vi "Handle Error.vi"(8 "error in (no error)":errorcluster, 11 "uService Template in":refnum<class "Father of all uServices.lvclass">) -> (0 "error out":errorcluster, 2 "stop actor?":bool=TRUE, 3 "uService Template out":refnum<class "Father of all uServices.lvclass">)   [LabVIEW 2026, in "TALOS.lvlib" / "Father of all uServices.lvlib" / "Father of all uServices.lvclass"]
doc: "(<B>Filename</B>: Actor Framework.lvlib:Actor.lvclass:Handle Error.vi)\n\nDefines how the actor handles an error that occurred while processing a message. By default, this method does nothing except stop the actor."
uses:
  Father of all uServices.lvclass
  <vilib>/Utility/error.llb/Error Cluster From Error Code.vi
  <vilib>/ErrorRing/Error Ring.xnode
  Ancestor/Ancestor/Ancestor.lvclass
  <vilib>/MultiError/TokenizeJSON/Multi Error Cluster.lvlib
  TALOS.lvlib
  Classes/Error Filter/Error Filter.lvclass
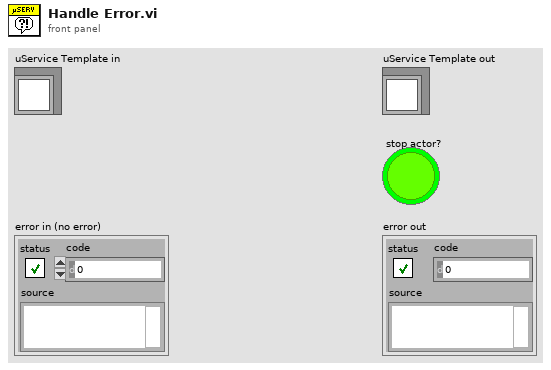
[diagram p1: front panel]
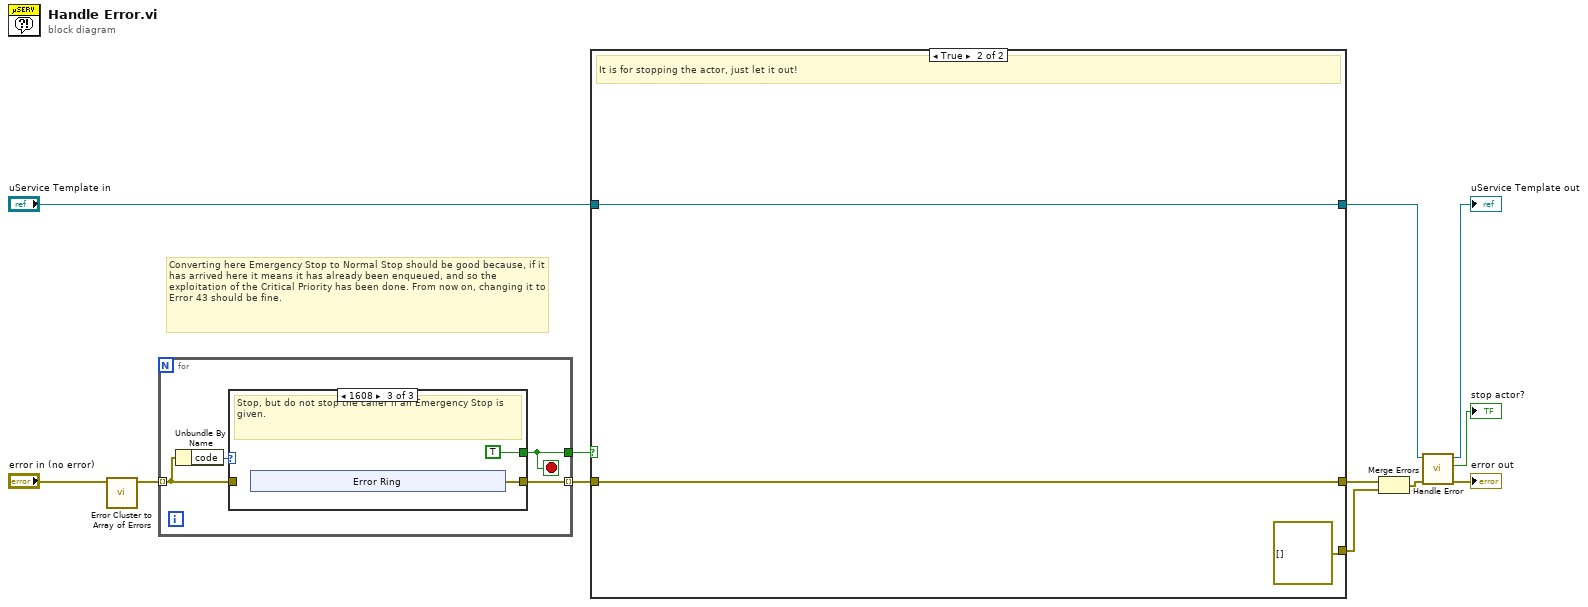
[diagram p0: block diagram]
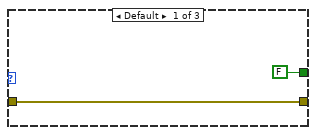
[diagram p2: hidden frame]
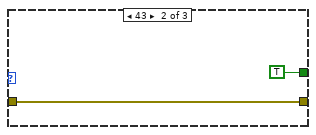
[diagram p3: hidden frame]
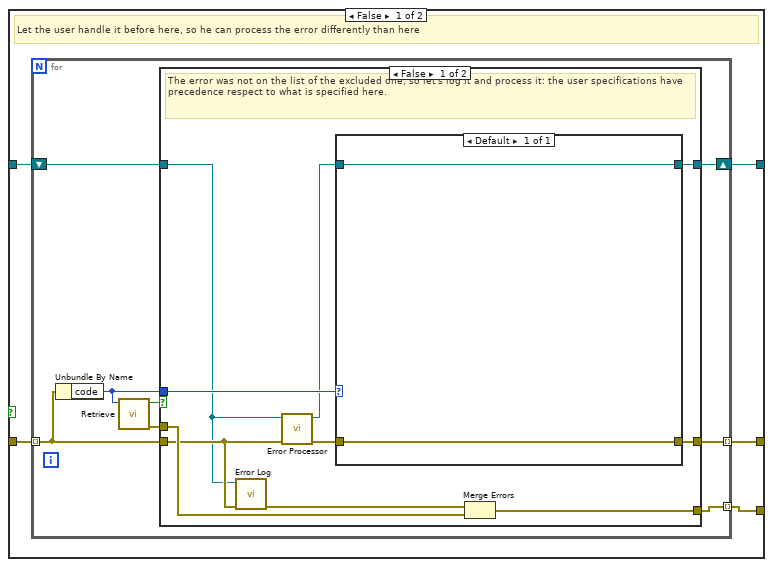
[diagram p4: hidden frame]
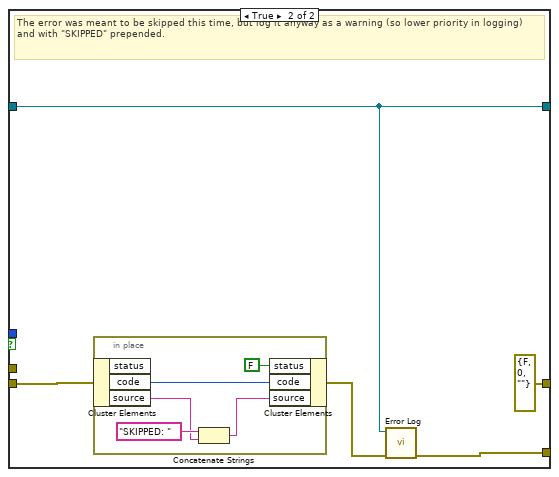
[diagram p5: hidden frame]
diagram:
  # "Converting here Emergency Stop to Normal Stop should be good because, if it has arrived here it means it has already been enqueued, and so the exploitation of the Critical Priority has been done. From now on, changing it to Error 43 should be fine."
  n1 = call <vilib>:"Error Cluster to Array of Errors.vi"("error"="error in (no error)") -> ("array of errors"=w8:errorcluster[])  [unwired: 10 in]
  n2 = for {
    tunnel: [w16] -> w4 mode=indexing
    tunnel: w8 -> [w13] mode=indexing
    tunnel: [w15] -> w5
    stop <- w15 stop-if-true
    n3 = Unbundle By Name(w13) -> ("code"=w14:i32)
    n4 = case shown="1608" w14 {
      tunnel: [w18 w20 w22] -> w16
      tunnel: w13 -> [w18 w20 _]
      tunnel: [FALSE TRUE TRUE] -> w15
      frame Default {
      }
      frame 43 {
      }
      frame 1608 {
        # "Stop, but do not stop the caller if an Emergency Stop is given."
        n5 = xnode "Error Ring"() -> ("error out"=w22:errorcluster)
      }
    }
  }
  n6 = case shown="True" w5 {
    tunnel: "uService Template in" -> [w31 w64]
    tunnel: [w29 w64] -> w6
    tunnel: w4 -> [w30 w63]
    tunnel: [w28 w63] -> w2
    tunnel: [w27 errorcluster[] [] ("error out")] -> w1
    frame False {
      # "Let the user handle it before here, so he can process the error differently than here"
      n7 = for {
        tunnel: w30 -> [w37] mode=indexing
        shift-right: [w38] -> w29
        shift-left: w31 -> [w36]
        tunnel: [w39] -> w28 mode=indexing
        tunnel: [w32] -> w27 mode=indexing
        n8 = Unbundle By Name(w37) -> ("code"=w35:i32)
        n9 = call "Retrieve.vi"("Error Code"=w35) -> ("error out"=w33:errorcluster, "Filter?"=w34:bool)  [unwired: 9 in]
        n10 = case shown="False" w34 {
          tunnel: [w48 errorcluster {"status"=FALSE, "code"=0, "source"=""} ("error out")] -> w39
          tunnel: [w47 w53] -> w38
          tunnel: w37 -> [w43 w55]
          tunnel: w36 -> [w42 w53]
          tunnel: w35 -> [w46 _]
          tunnel: [w40 w52] -> w32
          tunnel: w33 -> [w49 _]
          frame False {
            # "The error was not on the list of the excluded one, so let's log it and process it: the user specifications have precedence respect to what is specified here."
            n11 = call "Error Log.vi"("error in (no error)"=w43, "Object in"=w42) -> ("error out"=w41:errorcluster)  [unwired: 9 in]
            n12 = call-dynamic "Error Processor.vi"("error in (no error)"=w43, "Father of all uServices in"=w42) -> ("error out"=w45:errorcluster, "Father of all uServices out"=w44:refnum<class "Father of all uServices.lvclass">)  [unwired: 8 in]
            n13 = case shown="Default" w46 {
              tunnel: w45 -> [w50]
              tunnel: [w50] -> w48
              tunnel: w44 -> [w51]
              tunnel: [w51] -> w47
              frame Default {
              }
            }
            n14 = Merge Errors(w41, w49) -> (w40:errorcluster)
          }
          frame True {
            # "The error was meant to be skipped this time, but log it anyway as a warning (so lower priority in logging) and with \"SKIPPED\" prepended."
            n15 = in-place {
              n16 = in-place-cluster #1(w55) -> ("code"=w60:i32, "source"=w58:string)  [unwired: 1 out]
              n17 = Concatenate Strings("SKIPPED: " ("string"), w58) -> (w57:string)
              n18 = in-place-cluster #1("status"=FALSE, "code"=w60, "source"=w57) -> (w54:errorcluster)
            }
            n19 = call "Error Log.vi"("error in (no error)"=w54, "Object in"=w53) -> ("error out"=w52:errorcluster)  [unwired: 9 in]
          }
        }
      }
    }
    frame True {
      # "It is for stopping the actor, just let it out!"
    }
  }
  n20 = Merge Errors(w2, w1) -> (w3:errorcluster)
  n21 = call-parent "Handle Error.vi"("error in (no error)"=w3, "Ancestor in"=w6) -> ("error out"=→"error out":errorcluster, "stop actor?"=→"stop actor?":bool, "Ancestor out"=→"uService Template out":refnum<class "Father of all uServices.lvclass">)  [unwired: 7 in]
